vi "获取摄像头的video mode.vi"() -> ()   [LabVIEW 2017]
uses:
  <vilib>/userdefined/High Color/IMAQdx.ctl
  <vilib>/vision/driver/NI_Vision_Acquisition_Software.lvlib
panel:
  out "Current Mode":u32
  out "Video Modes":T1(array[cluster])
  in  "Camera Name":T2
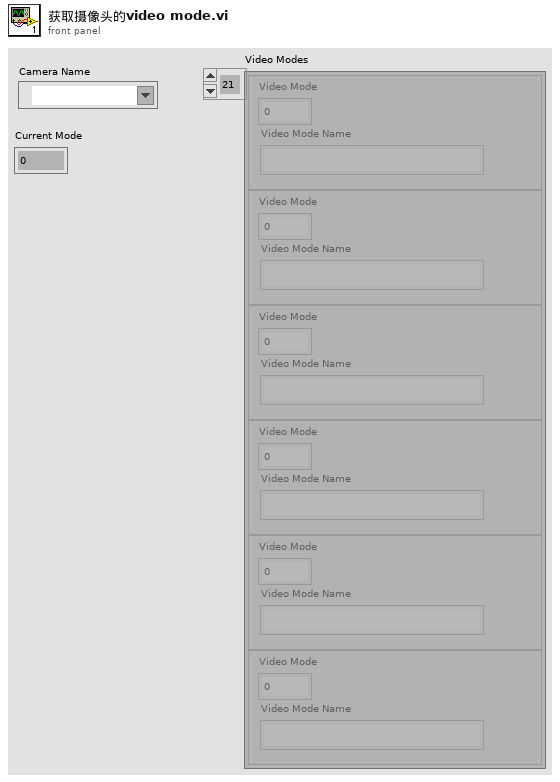
[diagram p1: front panel]
types:
  T1 = cluster{"Video Mode":u32, "Video Mode Name":string}[]
  T2 = typedef "IMAQdx.ctl" = refnum<k21>
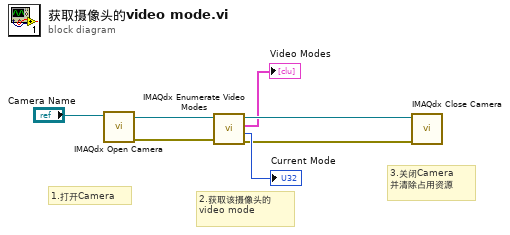
[diagram p0: block diagram]
diagram:
  # "2.获取该摄像头的\nvideo mode"
  # "3.关闭Camera\n并清除占用资源"
  # "1.打开Camera"
  n1 = call <vilib>:"IMAQdx Open Camera.vi"("Session In"="Camera Name") -> ("error out"=w5:errorcluster, "Session Out"=w6:T2)  [unwired: 2 in, 7 out]
  n2 = call <vilib>:"IMAQdx Enumerate Video Modes.vi"("error in"=w5, "Session In"=w6) -> ("error out"=w2:errorcluster, "Current Mode"=→"Current Mode":u32, "Video Modes"=→"Video Modes":T1, "Session Out"=w4:T2)  [unwired: 6 in]
  n3 = call <vilib>:"IMAQdx Close Camera.vi"("error in"=w2, "Session In"=w4) -> ()  [unwired: 10 out]
